vi "Force curl.vi"(0 "Vx":dbl, 1 "Vz":dbl, 2 "Vy":dbl, 3 "Instant_pos":dbl[](array[numeric]), 4 "current":u8, 5 "Type":u16) -> (6 "Fx":dbl, 7 "Fy":dbl, 8 "Fz":dbl)   [LabVIEW 2012]
uses:
  Global_var.vi
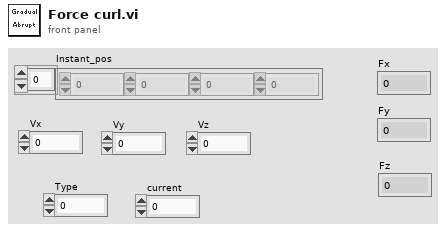
[diagram p1: front panel]
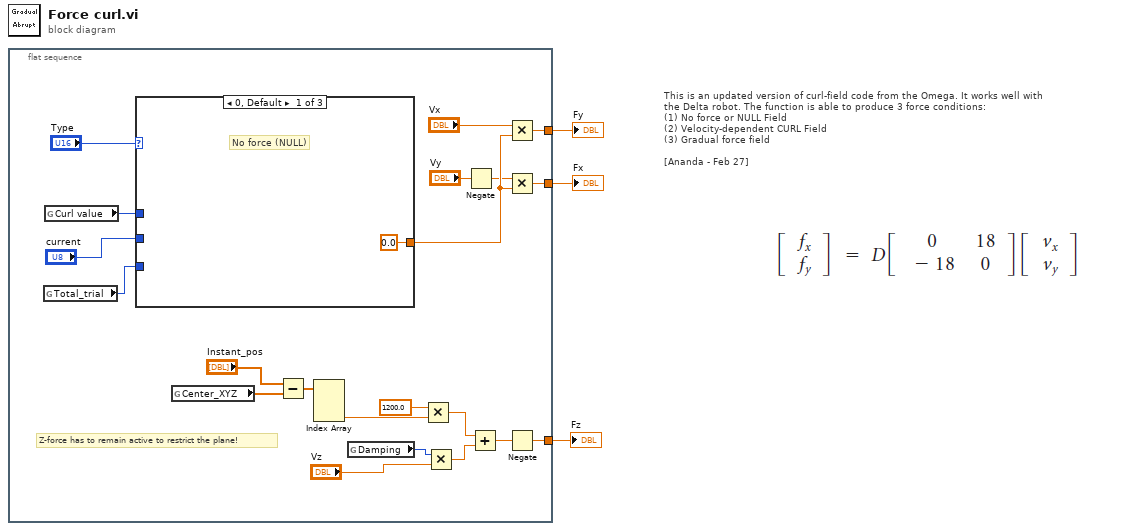
[diagram p0: block diagram]
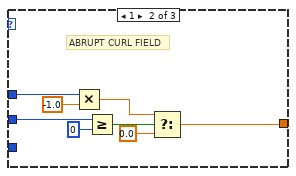
[diagram p2: hidden frame]
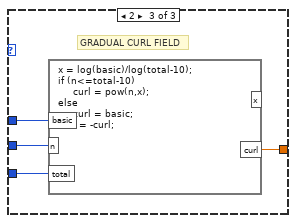
[diagram p3: hidden frame]
diagram:
  # "This is an updated version of curl-field code from the Omega. It works well with \nthe Delta robot. The function is able to produce 3 force conditions:\n(1) No force or NULL Field\n(2) Velocity-dependent CURL Field\n(3) Gradual force field\n\n[Ananda - Feb 27]"
  n1 = flat-sequence {
    tunnel: [w22] -> w3
    tunnel: [w9] -> w2
    tunnel: [w8] -> w1
    frame #0 {
      # "Z-force has to remain active to restrict the plane!"
      n2 = global read "Global_var.vi" "Total_trial"() -> (w12:u8)
      n3 = global read "Global_var.vi" "Curl value"() -> (w20:i8)
      n4 = case shown="0, Default" "Type" {
        tunnel: w20 -> [_ w28 w37]
        tunnel: [0.0 ("curl") w29 w36] -> w19
        tunnel: "current" -> [_ w33 w35]
        tunnel: w12 -> [_ _ w34]
        frame 0, Default {
          # "No force (NULL)"
        }
        frame 1 {
          # "ABRUPT CURL FIELD"
          n5 = Multiply(x=w28, y=-1.0) -> (x*y=w27:dbl)
          n6 = Greater Or Equal?(x=w33, y=u8 0) -> (x >= y?=w31:bool)
          n7 = Select(t=w27, s=w31, f=0.0) -> (s? t:f=w29:dbl)
        }
        frame 2 {
          # "GRADUAL CURL FIELD"
          n8 = formula code="x = log(basic)/log(total-10);\nif (n<=total-10)\n     curl = pow(n,x);\nelse\n     curl = basic;\ncurl = -curl;"("basic"=w37, "n"=w35, "total"=w34) -> ("curl"=w36:dbl)  [unwired: 1 out]
        }
      }
      n9 = global read "Global_var.vi" "Center_XYZ"() -> (w15:dbl[])
      n10 = Subtract(x="Instant_pos", y=w15) -> (x-y=w23:dbl[])
      n11 = Index Array(array=w23) -> (element #3=w21:dbl)  [unwired: 3 in, 2 out]
      n12 = global read "Global_var.vi" "Damping"() -> (w10:i16)
      n13 = Multiply(x=1200.0, y=w21) -> (x*y=w17:dbl)
      n14 = Multiply(x=w10, y="Vz") -> (x*y=w18:dbl)
      n15 = Negate(x="Vy") -> (-x=w7:dbl)
      n16 = Add(x=w17, y=w18) -> (x+y=w16:dbl)
      n17 = Multiply(x="Vx", y=w19) -> (x*y=w9:dbl)
      n18 = Multiply(x=w7, y=w19) -> (x*y=w8:dbl)
      n19 = Negate(x=w16) -> (-x=w22:dbl)
    }
  }
  "Fx" <- w1
  "Fy" <- w2
  "Fz" <- w3
